vi "RouteTrigSource.vi"(7 "Galil.IGalil":refnum<k7>, 8 "error in":errorcluster, 11 "Trig Source":u16(ring) items=["Function Gen Input", "Motion Trig", "Internal RT Motion Trig", "Internal CTR 1 Output"]) -> (0 "error out":errorcluster)   [LabVIEW 2022 SP3]
uses:
  Motion Controllers/Galil/Command Menu.ctl
  <vilib>/DAQmx/write.llb/DAQmx Write (Digital 1D Bool NChan 1Samp 1Line).vi
  <vilib>/DAQmx/miscellaneous.llb/DAQmx Fill In Error Info.vi
panel:
  in  "DAQ(t)/Galil(F)":bool=TRUE
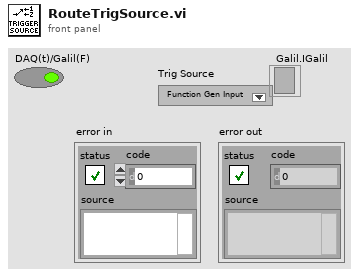
[diagram p1: front panel]
types:
  T1 = typedef "Command Menu.ctl" = enum16{"CommandPassThrough", "Abort Motion", "Define Pos", "Velocity", "Acceleration", "Deceleration", "Position Rel", "Postion Abs", "Begin Move", "After Move", "Home", "KI", "KD", "KP", "IL", "Config I/O", "Set Bit", "Clear Bit", "Motor Off", "Moto On", "Status", "Execute", "Halt Execute", "HX Status", "Tell Velocity", "Check Motion", "BreakPoint", "Tell Position", "Current Code Line", "Tell Switches", "OC Force On", "OC Off", "Pos Soft Limit", "Rev Soft Limit"}
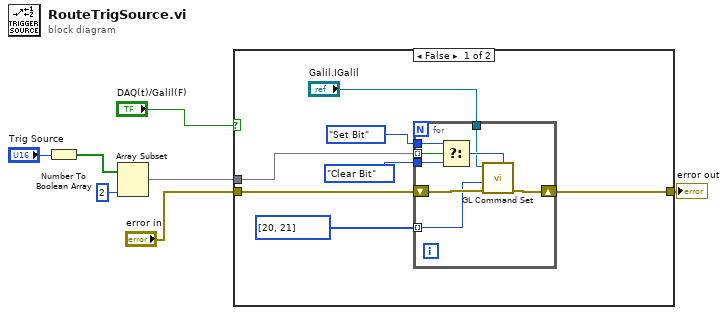
[diagram p0: block diagram]
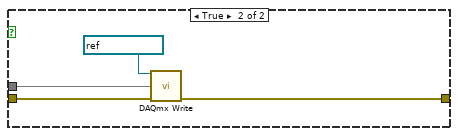
[diagram p2: hidden frame]
diagram:
  n1 = Number To Boolean Array(number="Trig Source") -> (Boolean array=w6:bool[])
  n2 = Array Subset(array=w6, length=2) -> (w5:bool[])  [unwired: 1 in]
  n3 = case shown="False" "DAQ(t)/Galil(F)" {
    tunnel: w5 -> [w12 w25]
    tunnel: [w14 w24] -> w3
    tunnel: "error in" -> [w13 w23]
    frame False {
      n4 = for {
        shift-right: [w22] -> w14
        shift-left: w13 -> [w21]
        tunnel: w12 -> [w19] mode=indexing
        tunnel: i32[] [20, 21] -> [w20] mode=indexing
        tunnel: Command_Menu."Set Bit" ("Command") -> [w18]
        tunnel: Command_Menu."Clear Bit" ("Command") -> [w17]
        tunnel: "Galil.IGalil" -> [w15]
        n5 = Select(t=w18, s=w19, f=w17) -> (s? t:f=w16:T1)
        n6 = call "GL Command Set.vi"("Command"=w16, "error in (no error)"=w21, "Value"=w20, "Galil.IGalil"=w15) -> ("error out"=w22:errorcluster)  [unwired: 3 in, 4 out]
      }
    }
    frame True {
      n7 = call-poly <vilib>:"DAQmx Write.vi"("task/channels in"=refnum<k21> "DIO-L2 L3", "data"=w25, "error in"=w23) -> ("error out"=w24:errorcluster)  [unwired: 10 in, 2 out]
    }
  }
  "error out" <- w3
